vi "joe_johnson_const.vi"() -> (3 "joe_johnson_const out":T1={"joe_johnson"={"joe_johnson_scale"={"min_ana"=0.0, "min_units"=0.0, "max_ana"=0.0, "max_units"=0.0}, "joe_johnson_idg"={"low_fault_ana"=0.0, "high_fault_ana"=0.0, "min_ana"=0.0, "max_ana"=0.0, "movement_thresh"=0.0, "movement_time"=0.0}, "joe_min_power"=0.0, "joe_motor_invert"=FALSE, "gain_scheduler"={"pid_min"={"kP"=0.0, "kI"=0.0, "kD"=0.0}, "pid_max"={"kP"=1.0, "kI"=0.1, "kD"=0.0}, "min"=0.0, "max"=1.0}, "max_integral"=0.0}})   [LabVIEW 2011]
uses:
  joe_johnson_const_t.ctl
  common/scale_const.ctl
  gun/gun_idg_const.ctl
  common/gain_sched_const.ctl
  common/gain_const.ctl
  Robot Global Data.vi
panel:
  in  "joe_johnson_const_practice":T1={"joe_johnson"={"joe_johnson_scale"={"min_ana"=4.44, "min_units"=0.0, "max_ana"=1.15, "max_units"=1.0}, "joe_johnson_idg"={"low_fault_ana"=4.8, "high_fault_ana"=0.6, "min_ana"=4.42, "max_ana"=1.2, "movement_thresh"=0.025, "movement_time"=250.0}, "joe_min_power"=0.15, "joe_motor_invert"=TRUE, "gain_scheduler"={"pid_min"={"kP"=1.12, "kI"=0.09, "kD"=0.0}, "pid_max"={"kP"=0.9, "kI"=0.1, "kD"=0.0}, "min"=0.0, "max"=0.8}, "max_integral"=0.7}}
  in  "joe_johnson_const_comp":T1={"joe_johnson"={"joe_johnson_scale"={"min_ana"=4.19, "min_units"=0.0, "max_ana"=1.24, "max_units"=1.0}, "joe_johnson_idg"={"low_fault_ana"=4.4, "high_fault_ana"=0.8, "min_ana"=4.22, "max_ana"=1.24, "movement_thresh"=0.025, "movement_time"=250.0}, "joe_min_power"=0.15, "joe_motor_invert"=TRUE, "gain_scheduler"={"pid_min"={"kP"=1.12, "kI"=0.09, "kD"=0.0}, "pid_max"={"kP"=0.9, "kI"=0.1, "kD"=0.0}, "min"=0.0, "max"=0.8}, "max_integral"=0.7}}
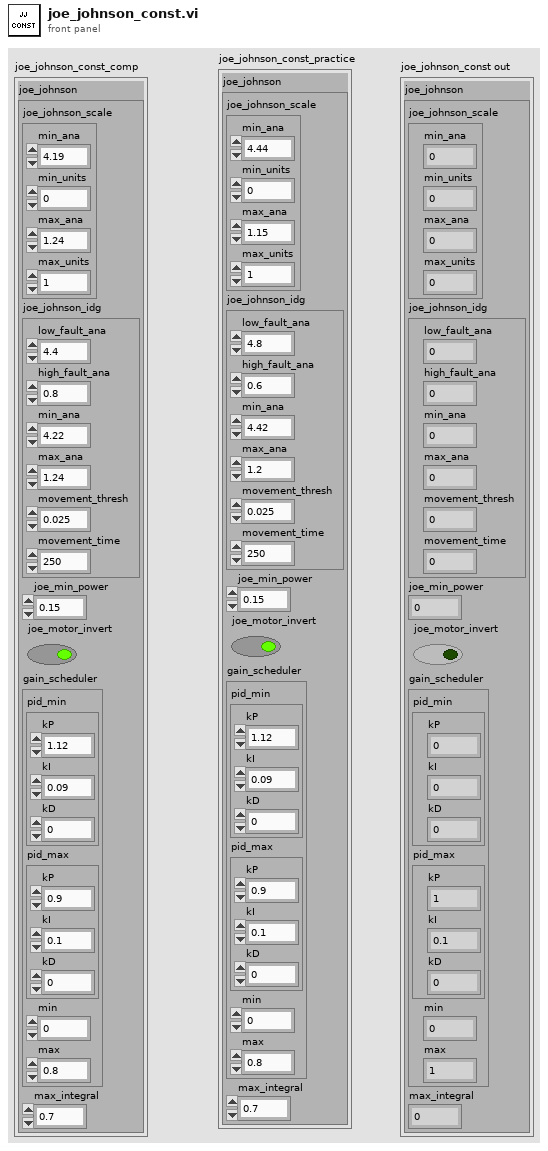
[diagram p1: front panel]
types:
  T1 = typedef "joe_johnson_const_t.ctl" = cluster{"joe_johnson":cluster{"joe_johnson_scale":T2, "joe_johnson_idg":T3, "joe_min_power":dbl, "joe_motor_invert":bool, "gain_scheduler":T4, "max_integral":dbl}}
  T2 = typedef "scale_const.ctl" = cluster{"min_ana":dbl, "min_units":dbl, "max_ana":dbl, "max_units":dbl}
  T3 = typedef "gun_idg_const.ctl" = cluster{"low_fault_ana":dbl, "high_fault_ana":dbl, "min_ana":dbl, "max_ana":dbl, "movement_thresh":dbl, "movement_time":dbl}
  T4 = typedef "gain_sched_const.ctl" = cluster{"pid_min":T5, "pid_max":T5, "min":dbl, "max":dbl}
  T5 = typedef "gain_const.ctl" = cluster{"kP":dbl, "kI":dbl, "kD":dbl}
  T6 = typedef "Robot Ctl.ctl" = enum16{"Competition", "Practice"}
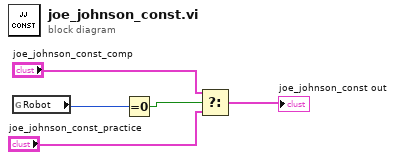
[diagram p0: block diagram]
diagram:
  n1 = global read "Robot Global Data.vi" "Robot"() -> (w5:T6)
  n2 = Equal To 0?(x=w5) -> (x = 0?=w3:bool)
  n3 = Select(t="joe_johnson_const_comp", s=w3, f="joe_johnson_const_practice") -> (s? t:f=→"joe_johnson_const out":T1)
